vi "Save-Load Initial Values-ROI entry window.vi"(6 "Which file? (User profile.ini)":T1=enum."Loaded User profile.ini", 8 "error in":errorcluster, 11 "Function":T2=enum."Load from file") -> (0 "error out":errorcluster)   [LabVIEW 2017]
uses:
  Typedefs/Save-Load enum.ctl
  Typedefs/Which path.ctl
  <vilib>/Utility/config.llb/NI_LVConfig.lvlib
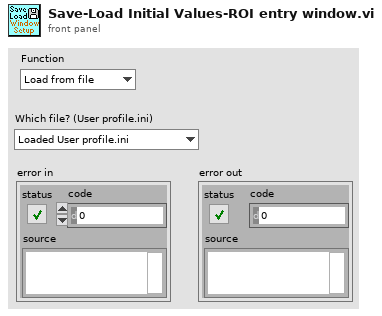
[diagram p1: front panel]
types:
  T1 = typedef "Which path.ctl" = enum16{"Configuration Files", "Calibration Files", "Images", "Setup.ini", "Loaded User profile.ini", "User's-Previous session.ini", "New user profile.ini", "Selected User profile.ini", "User profiles folder", "Power meter scaling.txt", "FOV Cal.ini"}
  T2 = typedef "Save-Load enum.ctl" = enum16{"Save to file", "Load from file", "Compare from file"}
  T3 = typedef "Ini file interface (DBL).ctl" = cluster{"key":string, "Save?":bool, "Default":dbl}[]
  T4 = typedef "Ini file interface (String).ctl" = cluster{"key":string, "Save?":bool, "Default":string}[]
  T5 = typedef "Ini file interface (Boolean).ctl" = cluster{"key":string, "Save?":bool, "Default":bool}[]
  T6 = typedef "NI_LVConfig.lvlib/Config Data RefNum.ctl" = refnum<k1>
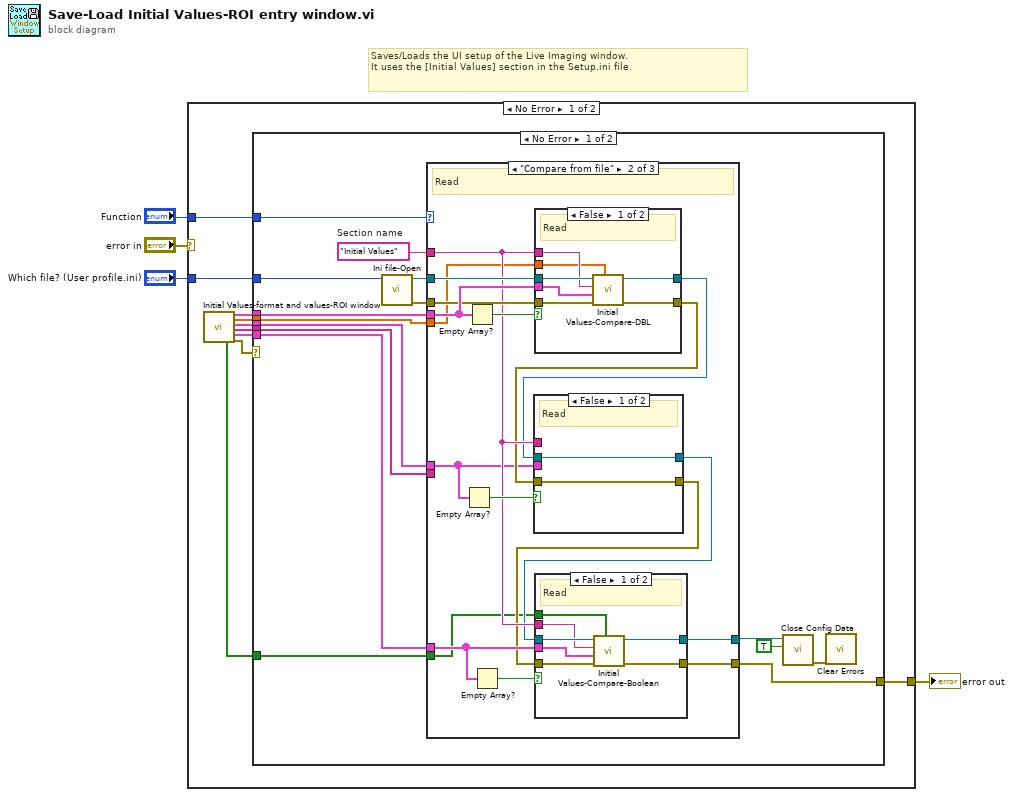
[diagram p0: block diagram]
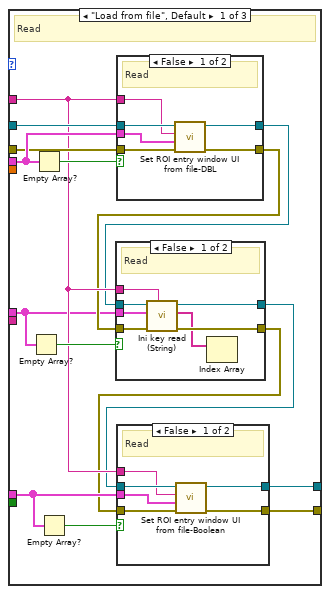
[diagram p2: hidden frame]
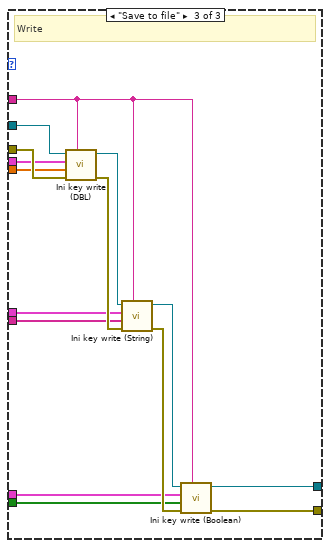
[diagram p9: hidden frame]
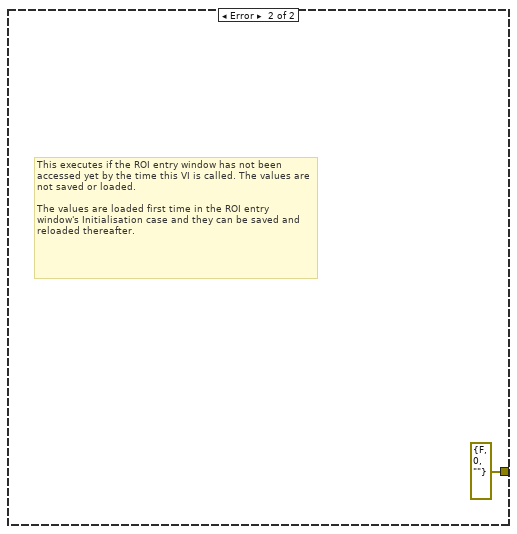
[diagram p10: hidden frame]
diagram:
  # "Saves/Loads the UI setup of the Live Imaging window.\nIt uses the [Initial Values] section in the Setup.ini file."
  n1 = case shown="No Error" "error in" {
    selector: "error in" -> [_ w125]
    tunnel: [w14 w125] -> w4
    tunnel: "Function" -> [w8 _]
    tunnel: "Which file? (User profile.ini)" -> [w5 _]
    frame No Error {
      n2 = call "Initial Values-format and values-ROI window.vi"() -> ("Values.Boolean"=w7:bool[], "Keys setup.DBL"=w13:T3, "Values.DBL"=w12:dbl[], "Keys setup.String"=w11:T4, "Values.Strings"=w10:string[], "Keys setup.Boolean"=w9:T5, "error out"=w6:errorcluster)  [unwired: 13 in]
      n3 = case shown="No Error" w6 {
        tunnel: [w23 errorcluster {"status"=FALSE, "code"=0, "source"=""} ("error out")] -> w14
        tunnel: w13 -> [w22 _]
        tunnel: w12 -> [w21 _]
        tunnel: w11 -> [w20 _]
        tunnel: w10 -> [w19 _]
        tunnel: w9 -> [w18 _]
        tunnel: w8 -> [w17 _]
        tunnel: w7 -> [w16 _]
        tunnel: w5 -> [w15 _]
        frame No Error {
          w29 = "Initial Values"  # Section name
          n4 = call "Ini file-Open.vi"("Which file?"=w15) -> ("error out"=w26:errorcluster, "User profile ini file ref"=w27:T6)  [unwired: 7 in, 2 out]
          n5 = case shown="\"Compare from file\"" w17 {
            tunnel: [w39 w81 w111] -> w23
            tunnel: [w40 w82 w110] -> w25
            tunnel: w26 -> [w41 w83 w122]
            tunnel: w27 -> [w44 w86 w123]
            tunnel: w29 -> [w35 w77 w113]
            tunnel: w22 -> [w43 w85 w120]
            tunnel: w21 -> [_ w71 w121]
            tunnel: w16 -> [_ w70 w112]
            tunnel: w18 -> [w38 w80 w114]
            tunnel: w19 -> [_ _ w117]
            tunnel: w20 -> [w30 w72 w109]
            frame "Load from file", Default {
              # "Read"
              n6 = Empty Array?(array=w30) -> (empty?=w36:bool)
              n7 = Empty Array?(array=w43) -> (empty?=w42:bool)
              n8 = Empty Array?(array=w38) -> (empty?=w37:bool)
              n9 = case shown="False" w42 {
                tunnel: w44 -> [w67 w69]
                tunnel: [w66 w69] -> w31
                tunnel: [w65 w68] -> w32
                tunnel: w41 -> [w64 w68]
                tunnel: w35 -> [w62 _]
                tunnel: w43 -> [w63 _]
                frame False {
                  # "Read"
                  n10 = call "Set ROI entry window UI from file-DBL.vi"("error in (no error)"=w64, "Keys setup.DBL"=w63, "Section name"=w62, "Refnum in"=w67) -> ("error out"=w65:errorcluster, "Refnum out"=w66:T6)  [unwired: 6 in]
                }
                frame True {
                  # "No parametersof such type"
                }
              }
              n11 = case shown="False" w36 {
                tunnel: [w48 w53] -> w34
                tunnel: [w47 w52] -> w33
                tunnel: w30 -> [w50 _]
                tunnel: w31 -> [w51 w53]
                tunnel: w32 -> [w46 w52]
                tunnel: w35 -> [w49 _]
                frame False {
                  # "Read"
                  n12 = call "Ini key read (String).vi"("Section name"=w49, "error in (no error)"=w46, "Keys setup"=w50, "Ini file ref in"=w51) -> ("error out"=w47:errorcluster, "Value read/used"=w45:string[], "Ini file ref"=w48:T6)  [unwired: 5 in]
                  n13 = Index Array(array=w45) -> ()  [unwired: 1 in, 1 out]
                }
                frame True {
                  # "No parametersof such type"
                }
              }
              n14 = case shown="False" w37 {
                tunnel: [w58 w61] -> w40
                tunnel: [w57 w60] -> w39
                tunnel: w38 -> [w54 _]
                tunnel: w34 -> [w59 w61]
                tunnel: w33 -> [w56 w60]
                tunnel: w35 -> [w55 _]
                frame False {
                  # "Read"
                  n15 = call "Set ROI entry window UI from file-Boolean.vi"("error in (no error)"=w56, "Keys setup.Boolean"=w54, "Section name"=w55, "Refnum in"=w59) -> ("error out"=w57:errorcluster, "Refnum out"=w58:T6)  [unwired: 6 in]
                }
                frame True {
                  # "No parametersof such type"
                }
              }
            }
            frame "Compare from file" {
              # "Read"
              n16 = Empty Array?(array=w72) -> (empty?=w78:bool)
              n17 = Empty Array?(array=w85) -> (empty?=w84:bool)
              n18 = Empty Array?(array=w80) -> (empty?=w79:bool)
              n19 = case shown="False" w84 {
                tunnel: w86 -> [w106 w108]
                tunnel: [w105 w108] -> w73
                tunnel: [w104 w107] -> w74
                tunnel: w83 -> [w103 w107]
                tunnel: w77 -> [w101 _]
                tunnel: w85 -> [w102 _]
                tunnel: w71 -> [w100 _]
                frame False {
                  # "Read"
                  n20 = call "Initial Values-Compare-DBL.vi"("Current values"=w100, "error in (no error)"=w103, "Keys Array"=w102, "Section name"=w101, "User profile ini file ref"=w106) -> ("error out"=w104:errorcluster, "User profile ini file ref"=w105:T6)  [unwired: 2 in, 3 out]
                }
                frame True {
                  # "No parametersof such type"
                }
              }
              n21 = case shown="False" w78 {
                tunnel: [w88 w90] -> w76
                tunnel: [w87 w89] -> w75
                tunnel: w72 -> [_ _]
                tunnel: w73 -> [w88 w90]
                tunnel: w74 -> [w87 w89]
                tunnel: w77 -> [_ _]
                frame False {
                  # "Read"
                }
                frame True {
                  # "No parametersof such type"
                }
              }
              n22 = case shown="False" w79 {
                tunnel: [w96 w99] -> w82
                tunnel: [w95 w98] -> w81
                tunnel: w80 -> [w92 _]
                tunnel: w76 -> [w97 w99]
                tunnel: w75 -> [w94 w98]
                tunnel: w77 -> [w93 _]
                tunnel: w70 -> [w91 _]
                frame False {
                  # "Read"
                  n23 = call "Initial Values-Compare-Boolean.vi"("Current values"=w91, "error in (no error)"=w94, "Keys Array"=w92, "Section name"=w93, "User profile ini file ref"=w97) -> ("error out"=w95:errorcluster, "User profile ini file ref"=w96:T6)  [unwired: 2 in, 3 out]
                }
                frame True {
                  # "No parametersof such type"
                }
              }
            }
            frame "Save to file" {
              # "Write"
              n24 = call "Ini key write (DBL).vi"("Section"=w113, "error in (no error)"=w122, "Values (DBL)"=w121, "Ini file interface"=w120, "Ini file refnum in"=w123) -> ("error out"=w118:errorcluster, "Ini file refnum out"=w119:T6)  [unwired: 5 in]
              n25 = call "Ini key write (String).vi"("Section"=w113, "error in (no error)"=w118, "Values (String)"=w117, "Ini file interface"=w109, "Ini file refnum in"=w119) -> ("error out"=w115:errorcluster, "Ini file refnum out"=w116:T6)  [unwired: 5 in]
              n26 = call "Ini key write (Boolean).vi"("Section"=w113, "error in (no error)"=w115, "Values (Boolean)"=w112, "Ini file interface"=w114, "Ini file refnum in"=w116) -> ("error out"=w111:errorcluster, "Ini file refnum out"=w110:T6)  [unwired: 5 in]
            }
          }
          n27 = call <vilib>:"Close Config Data.vi"("write file if changed (T)"=TRUE ("write configuration file? (F)"), "refnum"=w25) -> ("error out"=w24:errorcluster)  [unwired: 8 in, 1 out]
          n28 = call <vilib>:"Clear Errors.vi"("error in (no error)"=w24) -> ()  [unwired: 5 in, 2 out]
        }
        frame Error {
          # "This executes if the ROI entry window has not been accessed yet by the time this VI is called. The values are not saved or loaded.\n\nThe values are loaded first time in the ROI entry  window's Initialisation case and they can be saved and reloaded thereafter."
        }
      }
    }
    frame Error {
    }
  }
  "error out" <- w4
